vi "Enable-Disable UI Ctrls.vi"(6 "Controls":refnum<vi>[](array[refnum]), 7 "Disabled":T1(ring), 8 "error in (no error)":errorcluster) -> (0 "error out":errorcluster)   [LabVIEW 2017]
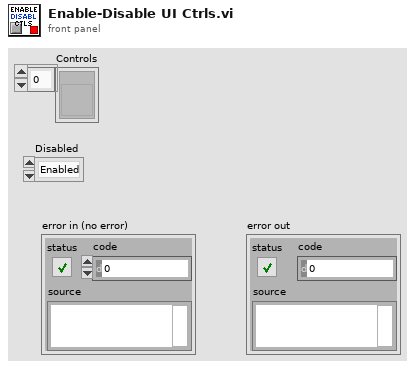
[diagram p1: front panel]
types:
  T1 = enum8{"Enabled", "Disabled", "Disabled and Grayed Out"}
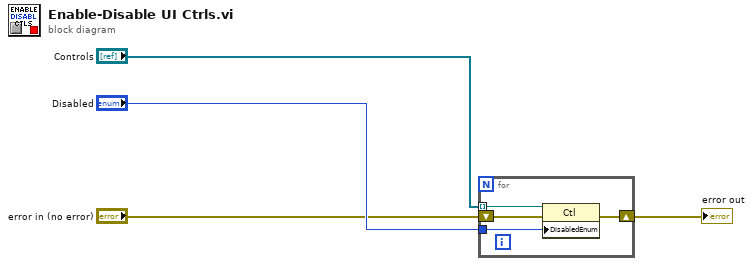
[diagram p0: block diagram]
diagram:
  n1 = for {
    shift-right: [w8] -> w4
    shift-left: "error in (no error)" -> [w7]
    tunnel: "Controls" -> [w6] mode=indexing
    tunnel: "Disabled" -> [w5]
    n2 = property class="Ctl"(reference=w6, error in=w7, "DisabledEnum"=w5) -> (error out=w8:errorcluster)  [unwired: 1 out]
  }
  "error out" <- w4
